vi "getNots.vi"(8 "error in (no error)":errorcluster, 11 "reference in":refnum<class "Notification Controller.lvclass">) -> (0 "error out":errorcluster, 1 "tracking_nots?":bool, 2 "nots?":bool, 3 "reference out":refnum<class "Notification Controller.lvclass">)   [LabVIEW 2016, in "Notification Controller.lvclass"]
uses:
  Notification Controller.lvclass
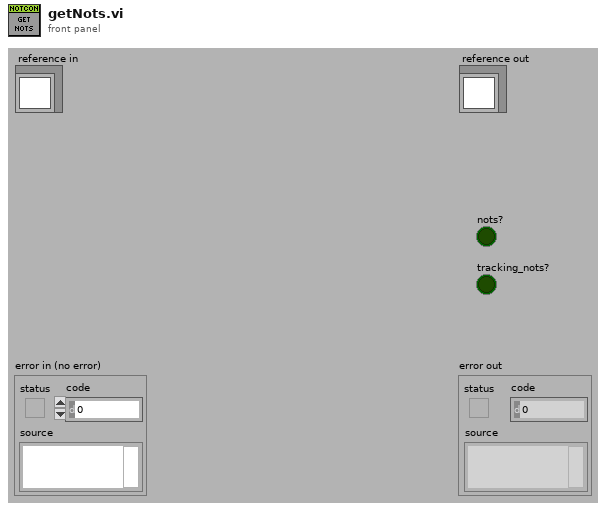
[diagram p1: front panel]
types:
  T1 = typedef "Notification Controller.lvclass/ObjectAttributesRef.ctl" = refnum<data-value>
  T2 = typedef "Notification Controller.lvclass/ObjectAttributes.ctl" = cluster{"MyAttribute":dbl, "items_data":string[][][], "items_notification_refs":refnum<class "itemsNotification.lvclass">[], "notifications_data_items":string[][], "items_nots?":bool, "devices_controller_ref":refnum<class "Devices Controller.lvclass">, "onlineUpdate":timestamp, "notController?":bool, "tracking_notification_ref":refnum<class "trackingNotification.lvclass">, "notifications_data_tracking":string[][], "tracking_parts_data":string[][], "tracking_nots?":bool, "index_tracking_not":i32[], "file_controller_ref":refnum<class "File Controller.lvclass">}
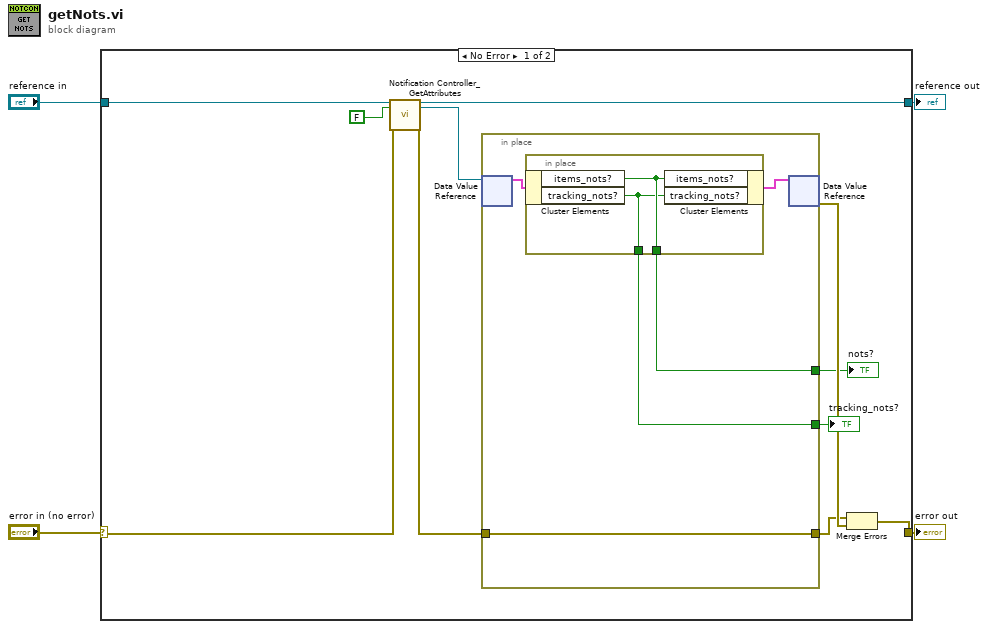
[diagram p0: block diagram]
diagram:
  n1 = case shown="No Error" "error in (no error)" {
    selector: "error in (no error)" -> [w10 w24]
    tunnel: [w15 w24] -> w3
    tunnel: [w8 w23] -> w1
    tunnel: "reference in" -> [w12 w23]
    frame No Error {
      n2 = call "Notification Controller_GetAttributes.vi"("reference in"=w12, "return data? (T)"=FALSE, "error in (no error)"=w10) -> ("reference out"=w8:refnum<class "Notification Controller.lvclass">, "attributes ref"=w7:T1, "error out"=w9:errorcluster)  [unwired: 13 in, 1 out]
      n3 = in-place {
        in-place-border: w9 -> [w18]
        in-place-border: [w18] -> w13
        in-place-border: [w17] -> w6
        in-place-border: [w16] -> w5
        n4 = in-place-dvr #1(w7) -> (w19:T2)  [unwired: 1 out]
        n5 = in-place {
          in-place-border: [w22] -> w17
          in-place-border: [w21] -> w16
          n6 = in-place-cluster #2(w19) -> ("items_nots?"=w22:bool, "tracking_nots?"=w21:bool)
          n7 = in-place-cluster #2("items_nots?"=w22, "tracking_nots?"=w21) -> (w20:T2)
        }
        n8 = in-place-dvr #1(w20) -> (w14:errorcluster)  [unwired: 1 out]
      }
      "nots?" <- w6
      "tracking_nots?" <- w5
      n9 = Merge Errors(w13, w14) -> (w15:errorcluster)
    }
    frame Error {
    }
  }
  "error out" <- w3
  "reference out" <- w1
